vi "Complete Measurament RT.vi"() -> ()   [LabVIEW 2014]
uses:
  <vilib>/Platform/TimedLoop/XDataNode/timing_clust.ctl
  <vilib>/Platform/TimedLoop/XDataNode/nitl_modes.ctl
  <vilib>/Platform/TimedLoop/XDataNode/wakeup.ctl
  <vilib>/Analysis/Matrix/Datatypes/RealMatrix.ctl
  <vilib>/FPGAPlugInAG/sbRIO-9636/niLvFpga_Open_sbRIO-9636.vi
  <vilib>/rvi/interface/common/dynamic/niFpgaDynamicAddResources.vi
  <vilib>/FPGAPlugInAG/Dynamic/niLvFpga_Reset_Dynamic.vi
  <vilib>/Utility/error.llb/Error Cluster From Error Code.vi
  <vilib>/rvi/errors/niLvFpgaAdjustHostInterfaceError.vi
  <vilib>/rvi/interface/common/niFpgaWaitOnOcc.vi
  <vilib>/FPGAPlugInAG/Dynamic/niLvFpga_Run_Dynamic.vi
  <vilib>/FPGAPlugInAG/Dynamic/niLvFpga_Abort_Dynamic.vi
  <vilib>/FPGAPlugInAG/Dynamic/niLvFpga_Close_Dynamic.vi
  <vilib>/rvi/interface/nirviOpenFPGA/nirviOpenFPGA.xnode
  FPGA Bitfiles/LaserDistanceSen_FPGATarget_N-ParametricDoub_YVLbjAYtdP4.lvbitx
  FPGA Target/Test VIs/N-Parametric Double FFT Mesurament Test.vi
  FPGA Bitfiles/LaserDistanceSen_FPGATarget_N-ParametricDoub_qx5IM88U9d4.lvbitx
  FPGA Target/Test VIs/N-Parametric Double FFT Mesurament Test SLOW.vi
  <vilib>/rvi/interface/nirviMethod/nirviMethod.xnode
  <vilib>/rvi/interface/nirviReadWriteControl/nirviReadWriteControl.xnode
  <vilib>/Platform/TimedLoop/XDataNode/XDataNode.xnode
  <vilib>/rvi/interface/nirviCloseFPGA/nirviCloseFPGA.xnode
  <vilib>/FPGAPlugInAG/Dynamic/niLvFpga_ConfigureFifo_Dynamic.vi
  <vilib>/rvi/errors/niLvFpgaMergeErrorWithErrorCode.vi
  <vilib>/FPGAPlugInAG/Dynamic/niLvFpga_StartFifo_Dynamic.vi
  <vilib>/rvi/interface/Simulation/niFpgaSimulationCallBeginRW.vi
  <vilib>/FPGAPlugInAG/Dynamic/niLvFpga_ReadFifo_Dynamic.vi
  <vilib>/Platform/TimedLoop/XDataNode/XDNodeRunTimeDep.lvlib
  NiFpgaLv.dll
  <vilib>/Analysis/NI_AALBase.lvlib
  <vilib>/Analysis/Matrix/NI_Matrix.lvlib
panel:
  in  "Tab Control":enum32{"5 bin", "5 bin mean", "Distance "}(tab)
  out "5 bin FALL":T1(graph) caption="5 freq fall"
  out "5 bin RISE":T1(graph)
  out "5 bin mean/std FALL":T2(graph)
  in  "#meanBin":i32=100
  out "5 bin mean/std RISE":T2(graph)
  out "Distance and error":T1(graph)
  in  "Sample /Modulation Frequency":enum32{"40MHz/32KHz", "30MHz/24Khz"}(radio)
  in  "#movesignal":i32=10
  out "moving standard deviation rel":dbl format="%0.5f"
  out "moving mean":dbl format="%0.7f"
  out "StdDev Rel 1":dbl
  out "StdDev Rel 2":dbl
  out "Warning":bool
  out "Velocity (m/s)":dbl
  out "Distance (m)":dbl
  out "Mean Frequency":dbl
  out "Rise array size":i32
  out "Fall array size":i32
  out "Mean Frequency Rising (Hz)":dbl
  out "Mean Frequency Falling (Hz)":dbl
  in  "tieni premuto per":i32=1
  in  "Triangular Multiply Factor":dbl[](array[numeric])=[1.0, 0.8, 0.95, 0.85, 0.9]
  out "RISING Second Edge N-FFT":dbl[](graph)
  in  "Enable triangular scaling":bool=TRUE
  in  "Triangolo dritto?":bool
  out "FALLING First Edge N-FFT":dbl[](graph)
  in  "#Signals":u32(slide)=5 scale=1.0..5.0
  in  "stop":bool
  in  "Initial Latency points":u32(slide) scale=0.0..1249.0
  out "Elements Remaining FFT":u32
  out "Elements Remaining Signal":u32
  out "N-Signals":dbl[](graph)
  in  "Snapshot":bool
  in  "Windowing":T3(ring)=enum."Hanning"
  in  "first bin":i32=5
  in  "last bin":i32=255
  in  "lower limit 2":u32(slide)=738 scale=625.0..738.0
  in  "lower limit 1":u32(slide)=113 scale=0.0..113.0
  # "OFFLINE parameters"
  # "Max Detection FFT bin range"
  # "WARNING:\nOnce pressed wait untill the end of operation"
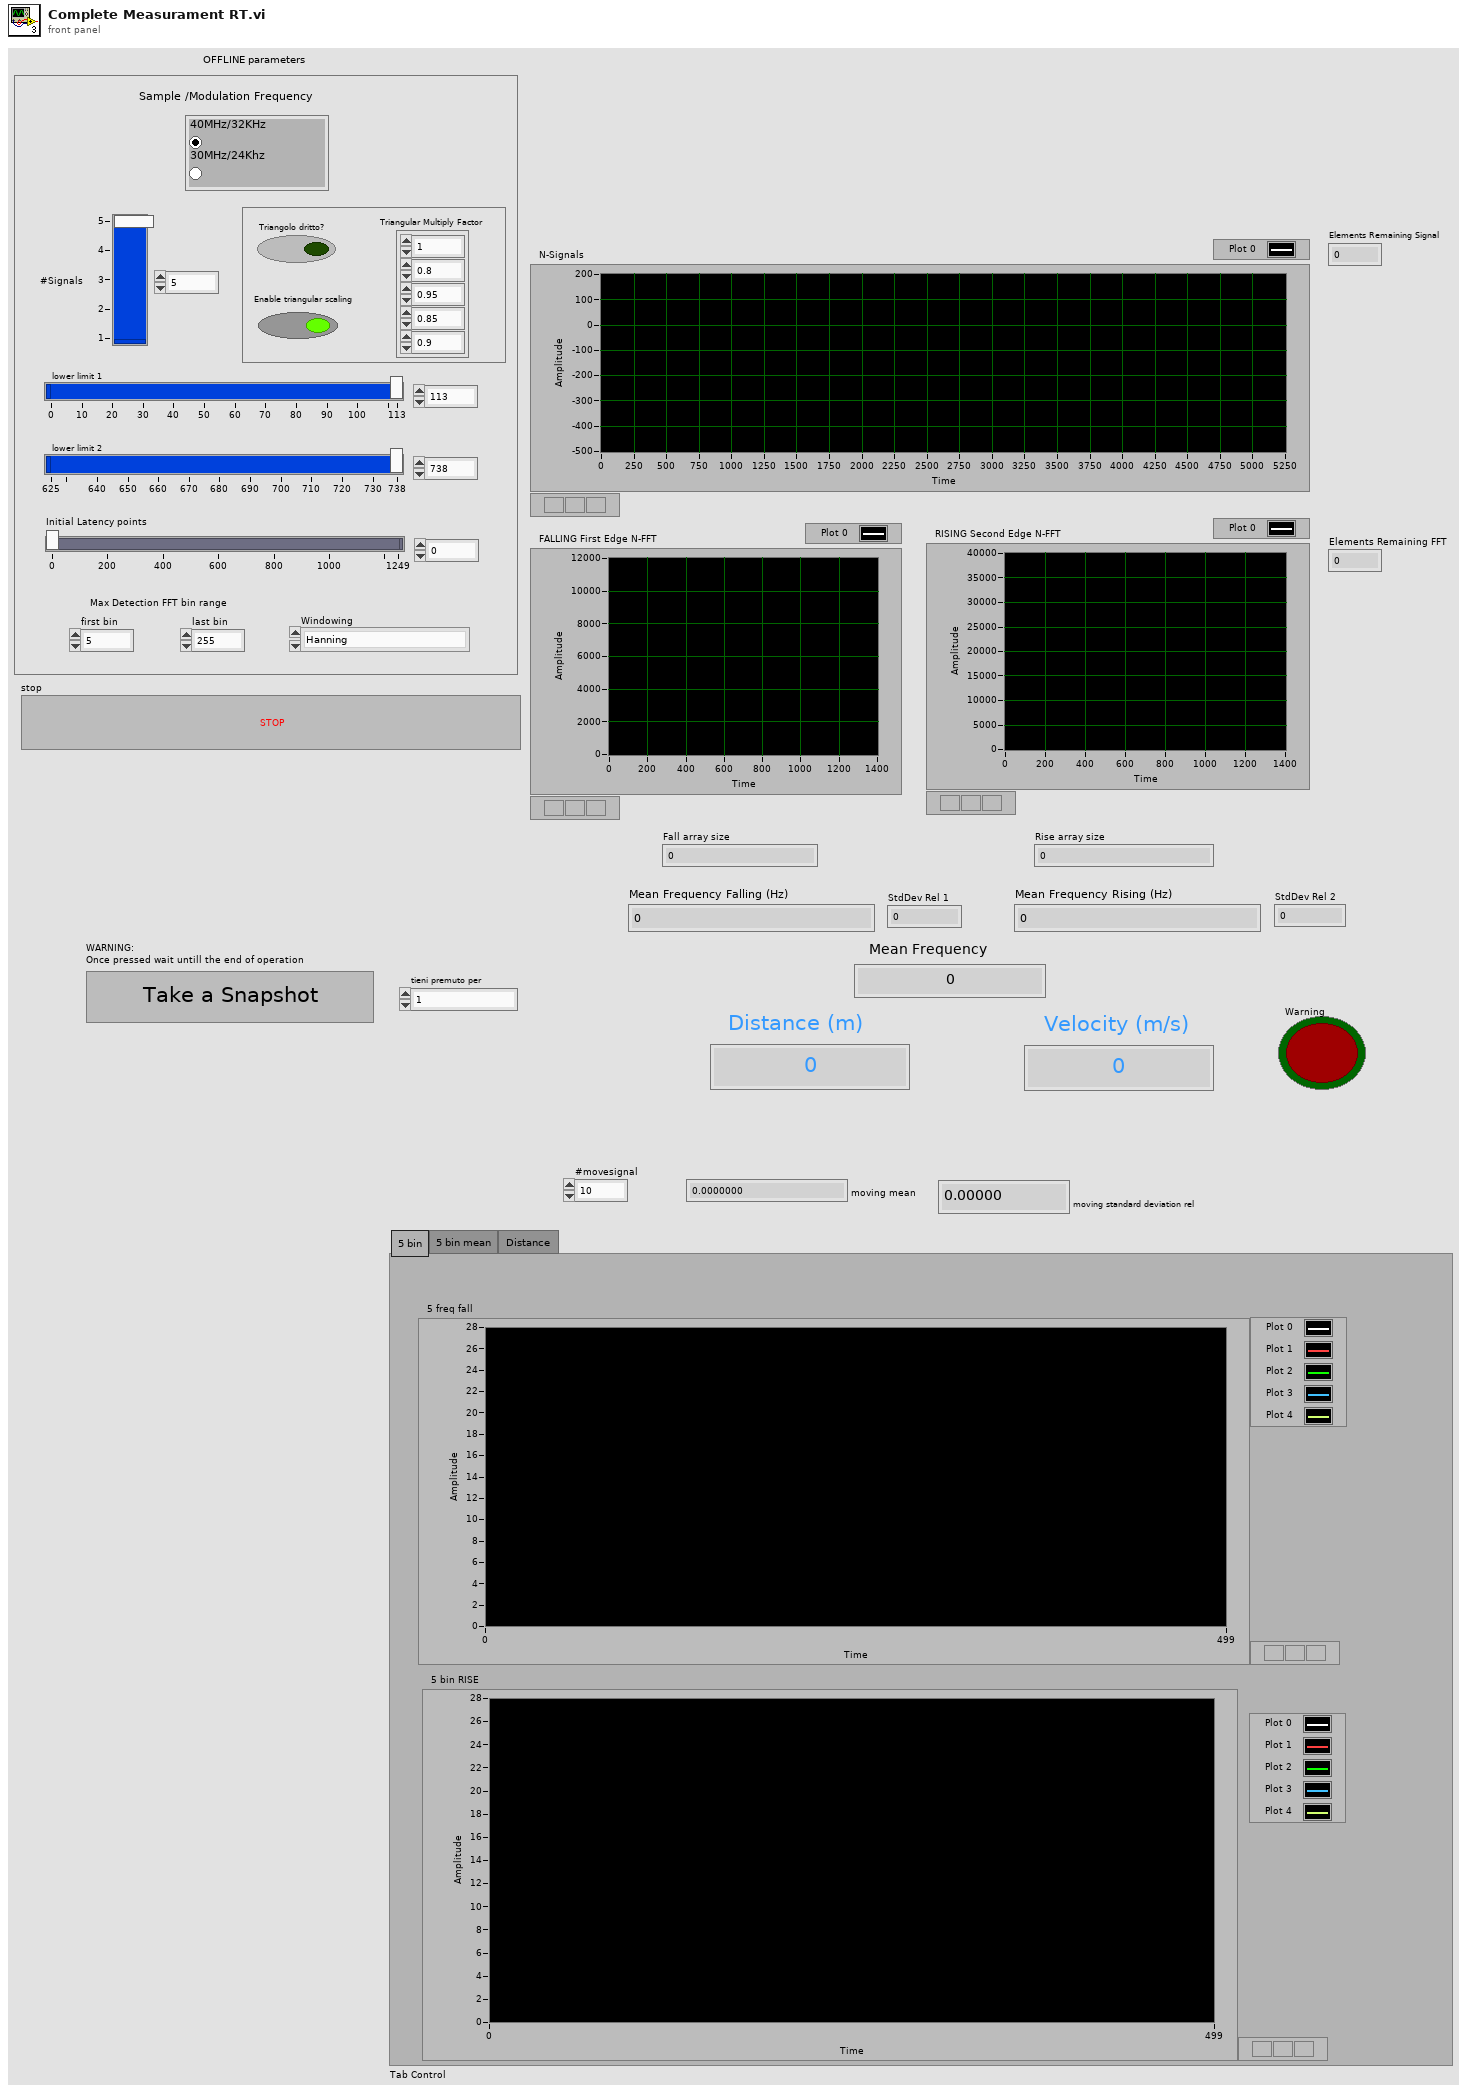
[diagram p1: front panel]
types:
  T1 = cluster{"[0]":dbl, "[1]":dbl, "[2]":dbl, "[3]":dbl, "[4]":dbl, "[5]":dbl, "[6]":dbl, "[7]":dbl, "[8]":dbl}
  T2 = cluster{"Array[0]":dbl, "Array[1]":dbl, "Array[2]":dbl, "Array[3]":dbl, "Array[4]":dbl, "Array[5]":dbl, "Array[6]":dbl, "Array[7]":dbl, "Array[8]":dbl}
  T3 = enum16{"None", "Hanning", "Hamming", "Blackman", "Blackman-Harris"}
  T4 = typedef "XDNodeRunTimeDep.lvlib/timing_clust.ctl" = cluster{"Expected End [f-1]":u64, "Actual End [f-1]":u64, "Finished Late? [f-1]":bool, "Expected End [i-1]":u64, "Actual End [i-1]":u64, "Finished Late? [i-1]":bool, "Expected Start [i]":u64, "Actual Start [i]":u64, "Expected Start [f]":u64, "Actual Start [f]":u64, "Source Name":string, "Structure Name":string, "Period":i64, "Deadline":i64, "Offset":i64, "Start":i64, "Priority":i32, "Timeout":i32, "Mode":T5, "Wakeup Reason":T6, "Error":errorcluster, "Source Type":string, "Secondary Source Type":string, "Global End Time":u64, "Global Start Time":u64, "Frame Duration":u64, "Iteration Duration":u64, "Assigned CPU":i32, "I/O Scan Engine Mode":u32}
  T5 = typedef "XDNodeRunTimeDep.lvlib/nitl_modes.ctl" = enum32{"No Change", "Process missed periods, maintain original phase", "Discard missed periods, maintain original phase", "Process missed periods, ignore original phase", "Discard missed periods, ignore original phase"}
  T6 = typedef "XDNodeRunTimeDep.lvlib/wakeup.ctl" = enum32{"Normal", "Aborted", "Asynchronous wakeup", "Timing source error", "Timed loop error", "Timeout"}
  T7 = typedef "NI_Matrix.lvlib/RealMatrix.ctl" = dbl[][]
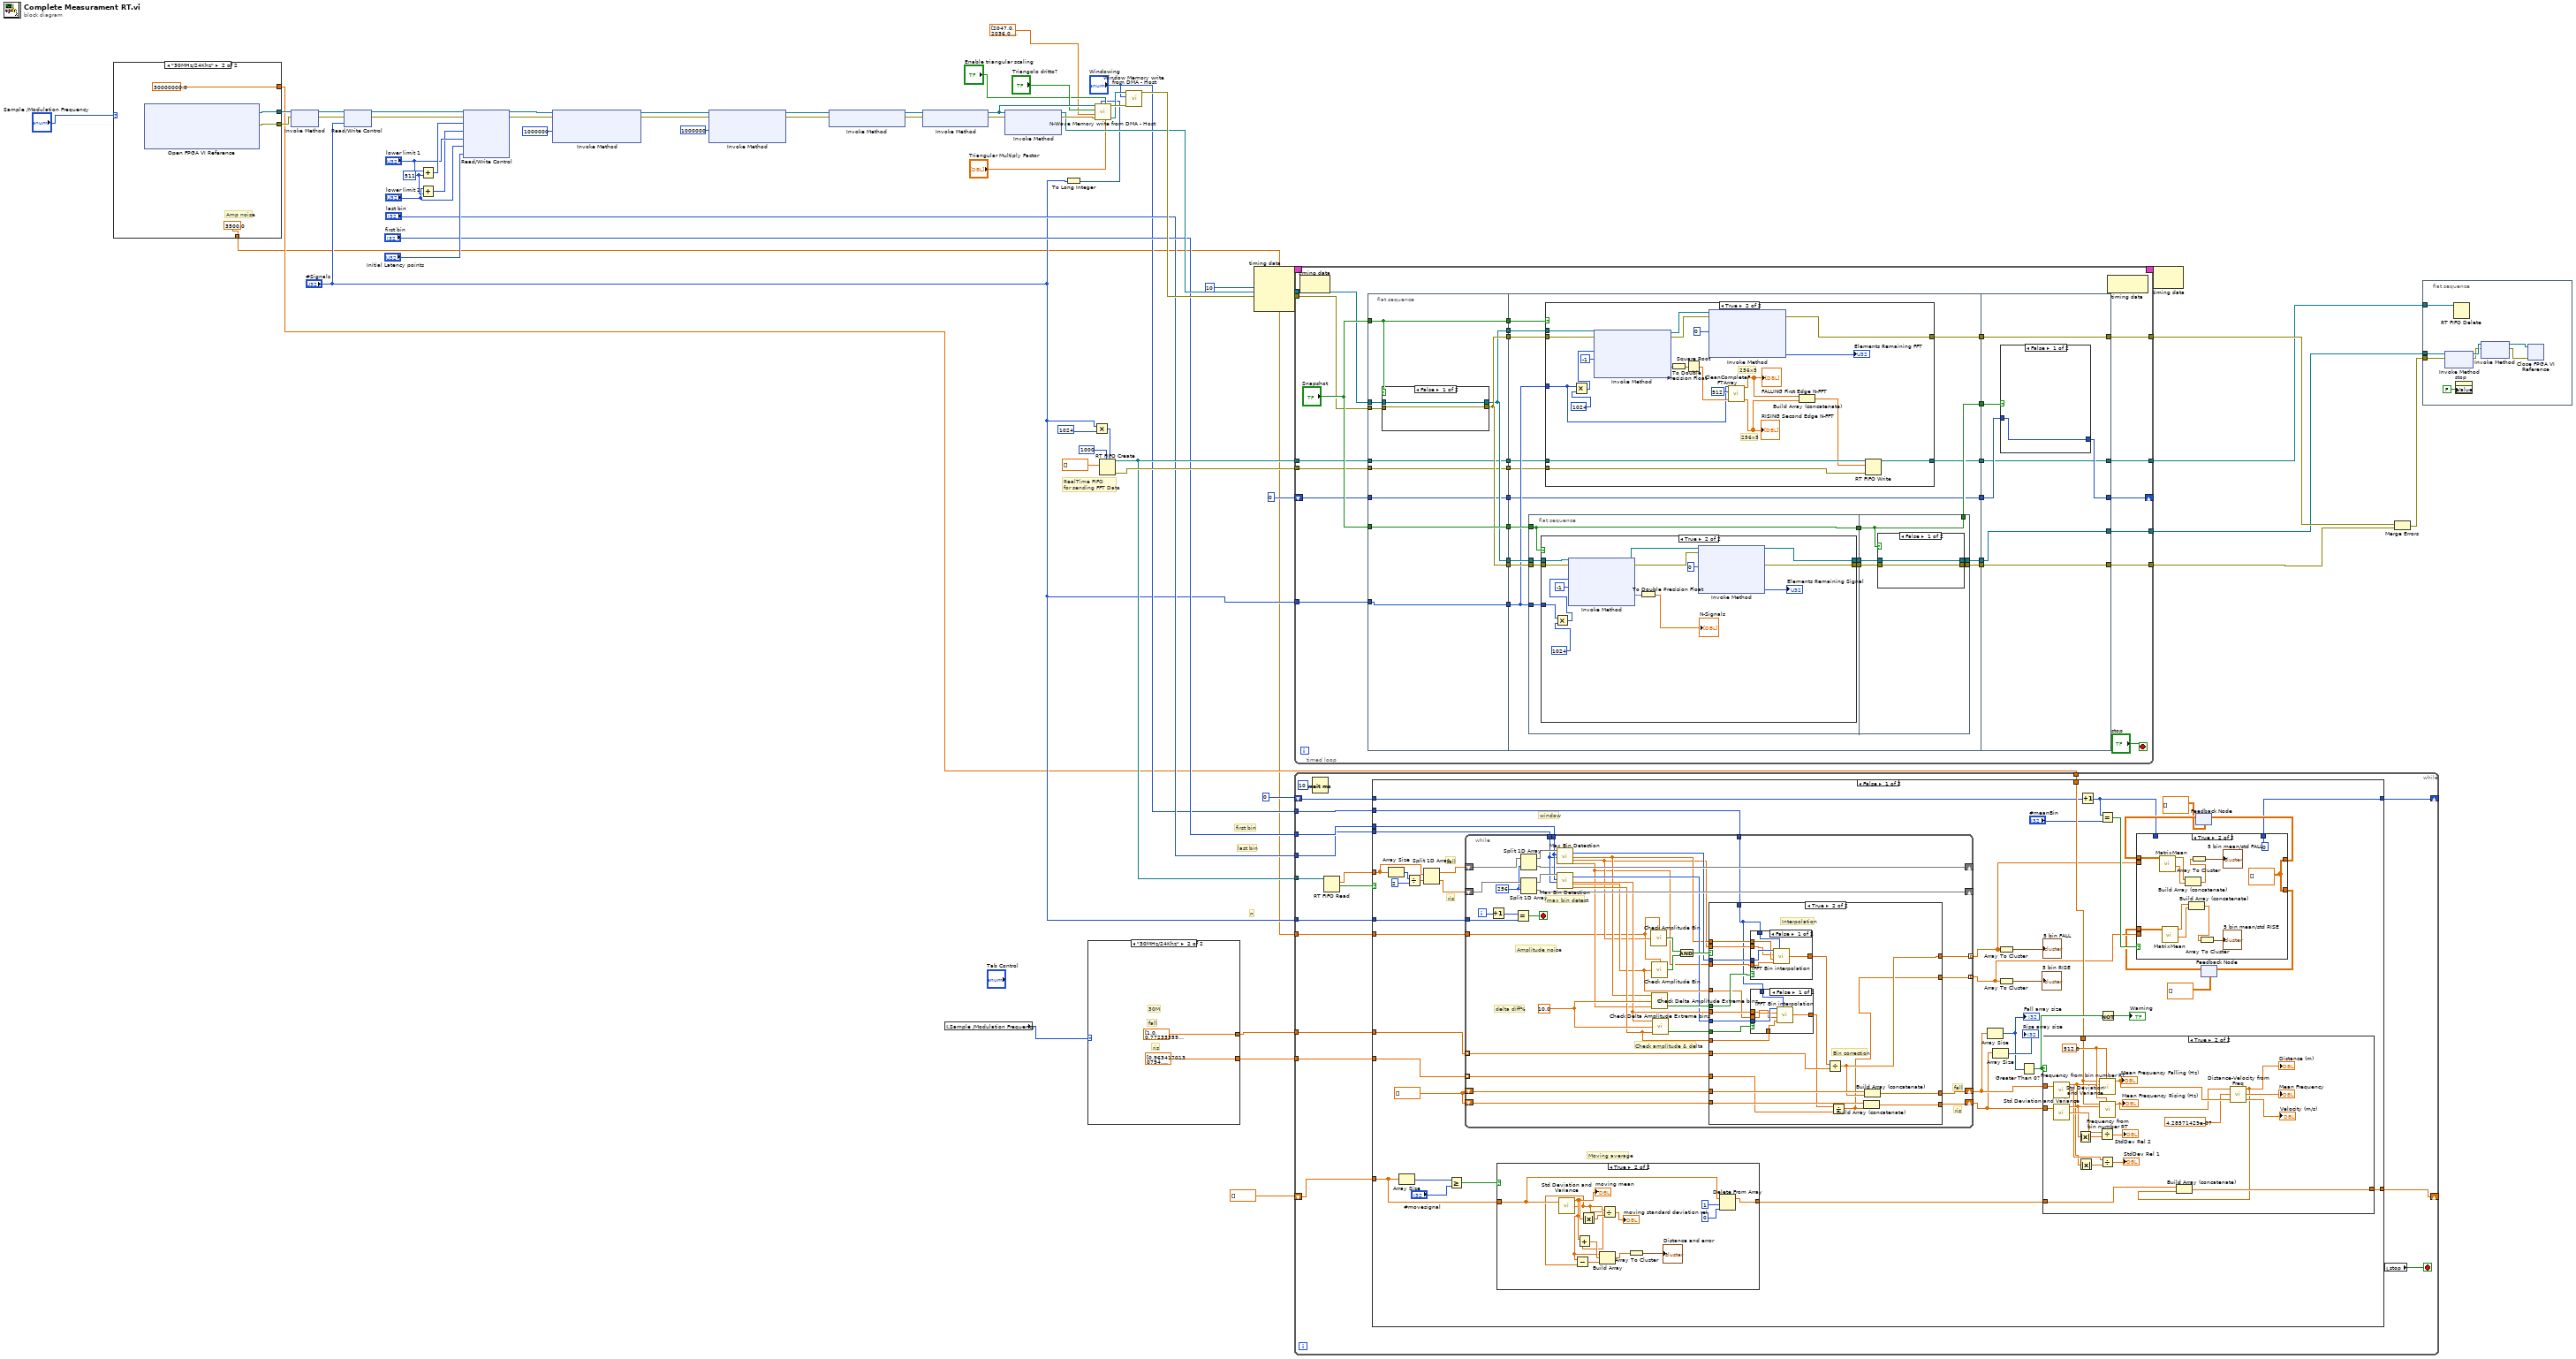
[diagram p0: block diagram]
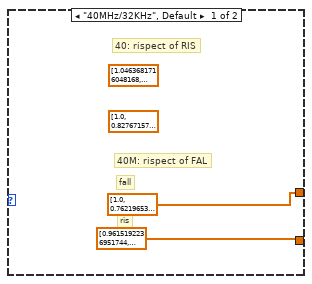
[diagram p2: hidden frame]
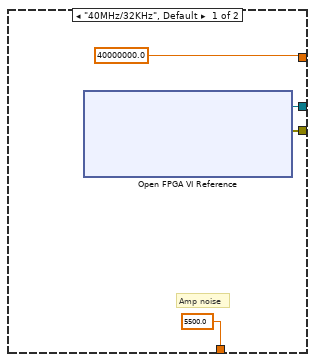
[diagram p3: hidden frame]
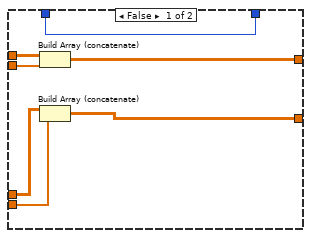
[diagram p4: hidden frame]
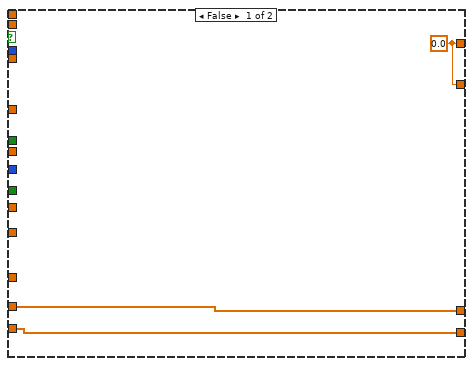
[diagram p7: hidden frame]
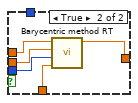
[diagram p8: hidden frame]
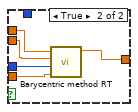
[diagram p9: hidden frame]
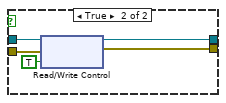
[diagram p11: hidden frame]
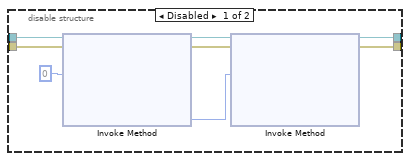
[diagram p13: hidden frame]
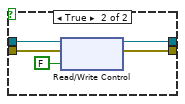
[diagram p14: hidden frame]
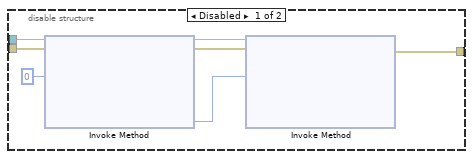
[diagram p16: hidden frame]
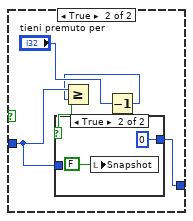
[diagram p17: hidden frame]
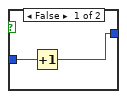
[diagram p18: hidden frame]
diagram:
  w57 = u32 511 ("y")
  # "n"
  # "last bin"
  # "first bin"
  # "RealTime FIFO \nfor sending FFT Data"
  n1 = case shown="\"30MHz/24Khz\"" "Sample /Modulation Frequency" {
    tunnel: [w65 w69] -> w31
    tunnel: [w64 w68] -> w30
    tunnel: [40000000.0 30000000.0] -> w6
    tunnel: [5500.0 ("Threshold Amp") 3500.0 ("Threshold Amp")] -> w1
    frame "40MHz/32KHz", Default {
      # "Amp noise"
      n2 = xnode "Open FPGA VI Reference"() -> ("FPGA VI Reference Out"=w65:refnum<k20>, "error out"=w64:errorcluster)  [unwired: 2 in]
    }
    frame "30MHz/24Khz" {
      # "Amp noise"
      n3 = xnode "Open FPGA VI Reference"() -> ("FPGA VI Reference Out"=w69:refnum<k20>, "error out"=w68:errorcluster)  [unwired: 2 in]
    }
  }
  n4 = xnode "Invoke Method"("FPGA VI Reference In"=w31, "error in"=w30) -> ("FPGA VI Reference Out"=w28:refnum<k20>, "error out"=w29:errorcluster)
  n5 = xnode "Read/Write Control"("FPGA VI Reference In"=w28, "error in"=w29, "n"="#Signals") -> ("FPGA VI Reference Out"=w27:refnum<k20>, "error out"=w26:errorcluster)
  n6 = Add(x="lower limit 1", y=w57) -> (x+y=w61:u32)
  n7 = Add(x="lower limit 2", y=w57) -> (x+y=w59:u32)
  n8 = xnode "Read/Write Control"("FPGA VI Reference In"=w27, "error in"=w26, "upper limit 1"=w61, "upper limit 2"=w59, "lower limit 1"="lower limit 1", "lower limit 2"="lower limit 2", "Latency points"="Initial Latency points") -> ("FPGA VI Reference Out"=w55:refnum<k20>, "error out"=w54:errorcluster)
  n9 = xnode "Invoke Method"("FPGA VI Reference In"=w55, "error in"=w54, "Requested Depth"=u32 1000000) -> ("FPGA VI Reference Out"=w42:refnum<k20>, "error out"=w43:errorcluster)  [unwired: 1 out]
  n10 = xnode "Invoke Method"("FPGA VI Reference In"=w42, "error in"=w43, "Requested Depth"=u32 1000000) -> ("FPGA VI Reference Out"=w49:refnum<k20>, "error out"=w50:errorcluster)  [unwired: 1 out]
  n11 = xnode "Invoke Method"("FPGA VI Reference In"=w49, "error in"=w50) -> ("FPGA VI Reference Out"=w40:refnum<k20>, "error out"=w41:errorcluster)
  n12 = xnode "Invoke Method"("FPGA VI Reference In"=w40, "error in"=w41) -> ("FPGA VI Reference Out"=w35:refnum<k20>, "error out"=w48:errorcluster)
  n13 = local read "Sample /Modulation Frequency"() -> (w3:enum32{"40MHz/32KHz", "30MHz/24Khz"})
  n14 = xnode "Invoke Method"("FPGA VI Reference In"=w35, "error in"=w48) -> ("FPGA VI Reference Out"=w36:refnum<k20>, "error out"=w39:errorcluster)  [unwired: 1 in]
  n15 = To Long Integer(number="#Signals") -> (32bit integer=w21:i32)
  n16 = case shown="\"30MHz/24Khz\"" w3 {
    tunnel: [dbl[] [1.0, 0.7621965374978185, 0.9584394857997629, 0.8264927572637538, 0.8956014637747813] ("mean factor 1") dbl[] [1.0, 0.7723335998303269, 0.9595435544705817, 0.8394441666056103, 0.8999330087703818] ("mean factor 1")] -> w5
    tunnel: [dbl[] [0.9615192236951744, 0.7991689735453839, 0.9195906148777597, 0.8398501694296071, 0.878805719221393] ("mean factor 2") dbl[] [0.9634170130794, 0.8025675631858347, 0.9199206430141584, 0.834350485116148, 0.8769354217012856] ("mean factor 2")] -> w4
    frame "40MHz/32KHz", Default {
      (unwired) dbl[] [1.0, 0.8276715727566772, 0.951057672906754, 0.8699894012780883, 0.9088749122499512] ("mean factor 2")
      (unwired) dbl[] [1.0463681716048168, 0.7798670577740541, 0.9941516729466621, 0.8518960261002109, 0.9344668620862013] ("mean factor 1")
      # "40: rispect of RIS"
      # "40M: rispect of FAL"
      # "ris"
      # "fall"
    }
    frame "30MHz/24Khz" {
      # "30M"
      # "ris"
      # "fall"
    }
  }
  n17 = Multiply(x="#Signals", y=u32 1024 ("elements in array (1)")) -> (x*y=w17:u32)
  n18 = call "N-Wave Memory write from DMA - Host.vi"("Triangular Multiply Factor"="Triangular Multiply Factor", "Enable triangular scaling"="Enable triangular scaling", "n"=w21, "error in"=w39, "Custom Triangular Signal (fal-ris)"=dbl[] [2047.0, 2036.0, 2024.0, 2013.0, 2002.0, 1990.0, 1979.0, 1968.0, 1956.0, 1945.0, 1934.0, 1923.0, 1912.0, 1900.0, 1889.0, 1878.0, 1867.0, 1856.0, 1845.0, 1833.0, 1822.0, 1811.0, 1800.0, 1789.0, 1778.0, 1767.0, 1756.0, 1745.0, 1734.0, 1723.0, 1712.0, 1702.0, 1691.0, 1680.0, 1669.0, 1658.0, 1647.0, 1636.0, 1626.0, 1615.0, 1604.0, 1593.0, 1583.0, 1572.0, 1561.0, 1550.0, 1540.0, 1529.0, 1518.0, 1508.0, 1497.0, 1487.0, 1476.0, 1465.0, 1455.0, 1444.0, 1434.0, 1423.0, 1413.0, 1402.0, 1392.0, 1381.0, 1371.0, 1360.0, 1350.0, 1340.0, 1329.0, 1319.0, 1309.0, 1298.0, 1288.0, 1278.0, 1267.0, 1257.0, 1247.0, 1237.0, 1226.0, 1216.0, 1206.0, 1196.0, 1186.0, 1176.0, 1165.0, 1155.0, 1145.0, 1135.0, 1125.0, 1115.0, 1105.0, 1095.0, 1085.0, 1075.0, 1065.0, 1055.0, 1045.0, 1035.0, 1025.0, 1015.0, 1006.0, 996.0, 986.0, 976.0, 966.0, 956.0, 947.0, 937.0, 927.0, 917.0, 908.0, 898.0, 888.0, 879.0, 869.0, 859.0, 850.0, 837.0, 826.0, 816.0, 804.0, 796.0, 788.0, 778.0, 769.0, 758.0, 750.0, 743.0, 733.0, 724.0, 717.0, 709.0, 701.0, 693.0, 686.0, 677.0, 669.0, 661.0, 653.0, 645.0, 638.0, 630.0, 622.0, 615.0, 607.0, 599.0, 592.0, 583.0, 576.0, 569.0, 561.0, 554.0, 547.0, 539.0, 532.0, 525.0, 518.0, 509.0, 501.0, 492.0, 486.0, 478.0, 471.0, 463.0, 456.0, 450.0, 442.0, 435.0, 429.0, 421.0, 415.0, 408.0, 401.0, 394.0, 388.0, 381.0, 375.0, 368.0, 361.0, 355.0, 349.0, 342.0, 336.0, 330.0, 323.0, 317.0, 311.0, 304.0, 298.0, 292.0, 286.0, 279.0, 273.0, 267.0, 261.0, 255.0, 249.0, 242.0, 236.0, 230.0, 224.0, 218.0, 212.0, 206.0, 200.0, 194.0, 187.0, 181.0, 175.0, 169.0, 163.0, 157.0, 150.0, 144.0, 138.0, 132.0, 125.0, 119.0, 113.0, 107.0, 101.0, 95.0, 88.0, 82.0, 77.0, 71.0, 65.0, 59.0, 53.0, 47.0, 41.0, 35.0, 29.0, 23.0, 18.0, 11.0, 6.0, 0.0, -6.0, -12.0, -18.0, -23.0, -29.0, -35.0, -41.0, -47.0, -52.0, -58.0, -64.0, -69.0, -75.0, -81.0, -87.0, -92.0, -98.0, -104.0, -109.0, -115.0, -121.0, -126.0, -132.0, -138.0, -144.0, -149.0, -155.0, -161.0, -166.0, -172.0, -177.0, -183.0, -189.0, -194.0, -200.0, -205.0, -211.0, -216.0, -222.0, -227.0, -233.0, -238.0, -244.0, -249.0, -255.0, -260.0, -266.0, -271.0, -277.0, -283.0, -288.0, -294.0, -299.0, -304.0, -310.0, -315.0, -321.0, -326.0, -331.0, -337.0, -342.0, -348.0, -353.0, -358.0, -364.0, -369.0, -375.0, -380.0, -385.0, -391.0, -396.0, -402.0, -407.0, -413.0, -418.0, -423.0, -429.0, -434.0, -439.0, -445.0, -450.0, -456.0, -461.0, -466.0, -472.0, -477.0, -483.0, -488.0, -493.0, -499.0, -504.0, -510.0, -515.0, -520.0, -526.0, -531.0, -537.0, -542.0, -548.0, -553.0, -558.0, -564.0, -569.0, -574.0, -580.0, -585.0, -590.0, -596.0, -601.0, -606.0, -612.0, -617.0, -622.0, -628.0, -633.0, -638.0, -644.0, -649.0, -654.0, -660.0, -665.0, -670.0, -676.0, -681.0, -686.0, -692.0, -697.0, -702.0, -708.0, -713.0, -718.0, -723.0, -729.0, -734.0, -739.0, -744.0, -750.0, -755.0, -760.0, -765.0, -771.0, -776.0, -781.0, -786.0, -792.0, -797.0, -802.0, -807.0, -812.0, -818.0, -823.0, -828.0, -833.0, -839.0, -844.0, -849.0, -854.0, -859.0, -865.0, -870.0, -875.0, -880.0, -885.0, -891.0, -896.0, -901.0, -906.0, -911.0, -916.0, -922.0, -927.0, -932.0, -937.0, -943.0, -948.0, -953.0, -958.0, -963.0, -969.0, -974.0, -979.0, -984.0, -989.0, -995.0, -1000.0, -1005.0, -1010.0, -1015.0, -1021.0, -1026.0, -1031.0, -1036.0, -1041.0, -1047.0, -1052.0, -1057.0, -1062.0, -1067.0, -1073.0, -1078.0, -1083.0, -1088.0, -1093.0, -1099.0, -1104.0, -1109.0, -1114.0, -1119.0, -1124.0, -1130.0, -1135.0, -1140.0, -1145.0, -1150.0, -1156.0, -1161.0, -1166.0, -1171.0, -1176.0, -1182.0, -1187.0, -1192.0, -1197.0, -1202.0, -1207.0, -1213.0, -1218.0, -1223.0, -1228.0, -1233.0, -1238.0, -1244.0, -1249.0, -1254.0, -1259.0, -1264.0, -1269.0, -1275.0, -1280.0, -1285.0, -1290.0, -1295.0, -1300.0, -1305.0, -1311.0, -1316.0, -1321.0, -1326.0, -1331.0, -1336.0, -1342.0, -1347.0, -1352.0, -1357.0, -1362.0, -1367.0, -1372.0, -1378.0, -1383.0, -1388.0, -1393.0, -1398.0, -1403.0, -1408.0, -1414.0, -1419.0, -1424.0, -1429.0, -1434.0, -1439.0, -1444.0, -1450.0, -1455.0, -1460.0, -1465.0, -1470.0, -1475.0, -1480.0, -1486.0, -1491.0, -1496.0, -1501.0, -1506.0, -1511.0, -1516.0, -1522.0, -1527.0, -1532.0, -1537.0, -1542.0, -1547.0, -1552.0, -1558.0, -1563.0, -1568.0, -1573.0, -1578.0, -1583.0, -1588.0, -1593.0, -1599.0, -1604.0, -1609.0, -1614.0, -1619.0, -1624.0, -1629.0, -1634.0, -1640.0, -1645.0, -1650.0, -1655.0, -1660.0, -1665.0, -1670.0, -1675.0, -1681.0, -1686.0, -1691.0, -1696.0, -1701.0, -1706.0, -1711.0, -1716.0, -1722.0, -1727.0, -1732.0, -1737.0, -1742.0, -1747.0, -1752.0, -1757.0, -1762.0, -1768.0, -1773.0, -1778.0, -1783.0, -1788.0, -1793.0, -1798.0, -1803.0, -1808.0, -1814.0, -1819.0, -1824.0, -1829.0, -1834.0, -1839.0, -1844.0, -1849.0, -1854.0, -1859.0, -1865.0, -1870.0, -1875.0, -1880.0, -1885.0, -1890.0, -1895.0, -1900.0, -1905.0, -1911.0, -1916.0, -1921.0, -1926.0, -1931.0, -1936.0, -1941.0, -1946.0, -1951.0, -1956.0, -1961.0, -1967.0, -1972.0, -1977.0, -1982.0, -1987.0, -1992.0, -1997.0, -2002.0, -2007.0, -2012.0, -2017.0, -2023.0, -2028.0, -2033.0, -2038.0, -2043.0, -2048.0, -2047.0, -2034.0, -2021.0, -2009.0, -1996.0, -1983.0, -1970.0, -1957.0, -1945.0, -1932.0, -1919.0, -1907.0, -1894.0, -1881.0, -1869.0, -1856.0, -1844.0, -1831.0, -1819.0, -1806.0, -1794.0, -1781.0, -1769.0, -1757.0, -1744.0, -1732.0, -1719.0, -1707.0, -1695.0, -1682.0, -1670.0, -1658.0, -1646.0, -1634.0, -1621.0, -1609.0, -1597.0, -1585.0, -1573.0, -1561.0, -1549.0, -1537.0, -1525.0, -1513.0, -1501.0, -1489.0, -1477.0, -1465.0, -1453.0, -1441.0, -1429.0, -1417.0, -1405.0, -1394.0, -1382.0, -1370.0, -1358.0, -1347.0, -1335.0, -1323.0, -1312.0, -1300.0, -1288.0, -1277.0, -1265.0, -1254.0, -1242.0, -1231.0, -1219.0, -1208.0, -1196.0, -1185.0, -1173.0, -1162.0, -1150.0, -1139.0, -1128.0, -1116.0, -1105.0, -1094.0, -1083.0, -1071.0, -1060.0, -1049.0, -1038.0, -1027.0, -1015.0, -1004.0, -993.0, -982.0, -971.0, -960.0, -949.0, -938.0, -927.0, -916.0, -905.0, -894.0, -883.0, -873.0, -862.0, -851.0, -840.0, -829.0, -819.0, -808.0, -797.0, -786.0, -776.0, -765.0, -754.0, -744.0, -733.0, -722.0, -712.0, -697.0, -685.0, -674.0, -661.0, -652.0, -643.0, -632.0, -622.0, -610.0, -602.0, -594.0, -583.0, -574.0, -566.0, -558.0, -550.0, -542.0, -534.0, -525.0, -516.0, -507.0, -499.0, -491.0, -483.0, -475.0, -467.0, -459.0, -451.0, -443.0, -435.0, -426.0, -419.0, -411.0, -404.0, -396.0, -388.0, -381.0, -373.0, -366.0, -359.0, -349.0, -341.0, -331.0, -325.0, -317.0, -309.0, -301.0, -295.0, -288.0, -280.0, -273.0, -266.0, -259.0, -252.0, -246.0, -239.0, -231.0, -225.0, -219.0, -212.0, -205.0, -199.0, -192.0, -186.0, -180.0, -173.0, -167.0, -161.0, -155.0, -148.0, -142.0, -136.0, -130.0, -124.0, -118.0, -112.0, -106.0, -100.0, -94.0, -88.0, -82.0, -76.0, -70.0, -64.0, -58.0, -52.0, -46.0, -40.0, -34.0, -28.0, -21.0, -15.0, -9.0, -3.0, 2.0, 9.0, 15.0, 21.0, 27.0, 33.0, 39.0, 45.0, 51.0, 57.0, 63.0, 69.0, 75.0, 81.0, 86.0, 92.0, 98.0, 103.0, 110.0, 116.0, 121.0, 127.0, 133.0, 138.0, 144.0, 149.0, 155.0, 161.0, 166.0, 172.0, 177.0, 183.0, 189.0, 194.0, 200.0, 205.0, 211.0, 216.0, 221.0, 227.0, 232.0, 238.0, 243.0, 249.0, 254.0, 259.0, 265.0, 270.0, 276.0, 281.0, 286.0, 292.0, 297.0, 303.0, 308.0, 314.0, 319.0, 324.0, 329.0, 335.0, 340.0, 345.0, 351.0, 356.0, 361.0, 366.0, 371.0, 377.0, 382.0, 387.0, 392.0, 397.0, 403.0, 408.0, 413.0, 418.0, 423.0, 429.0, 434.0, 439.0, 444.0, 449.0, 454.0, 459.0, 464.0, 469.0, 474.0, 479.0, 484.0, 489.0, 494.0, 499.0, 504.0, 509.0, 514.0, 520.0, 525.0, 530.0, 535.0, 540.0, 545.0, 550.0, 555.0, 560.0, 565.0, 570.0, 575.0, 580.0, 585.0, 590.0, 595.0, 600.0, 605.0, 610.0, 615.0, 620.0, 625.0, 630.0, 636.0, 641.0, 646.0, 651.0, 656.0, 661.0, 666.0, 671.0, 676.0, 681.0, 686.0, 691.0, 696.0, 701.0, 706.0, 711.0, 716.0, 721.0, 726.0, 731.0, 736.0, 741.0, 746.0, 751.0, 756.0, 761.0, 765.0, 770.0, 775.0, 780.0, 785.0, 790.0, 795.0, 800.0, 805.0, 810.0, 815.0, 820.0, 825.0, 829.0, 834.0, 839.0, 844.0, 849.0, 854.0, 859.0, 864.0, 868.0, 873.0, 878.0, 883.0, 888.0, 893.0, 897.0, 902.0, 907.0, 912.0, 917.0, 921.0, 926.0, 931.0, 936.0, 941.0, 945.0, 950.0, 955.0, 960.0, 965.0, 969.0, 974.0, 979.0, 984.0, 988.0, 993.0, 998.0, 1003.0, 1007.0, 1012.0, 1017.0, 1022.0, 1027.0, 1031.0, 1036.0, 1041.0, 1046.0, 1051.0, 1055.0, 1060.0, 1065.0, 1070.0, 1075.0, 1079.0, 1084.0, 1089.0, 1094.0, 1098.0, 1103.0, 1108.0, 1113.0, 1118.0, 1122.0, 1127.0, 1132.0, 1137.0, 1141.0, 1146.0, 1151.0, 1156.0, 1161.0, 1165.0, 1170.0, 1175.0, 1180.0, 1184.0, 1189.0, 1194.0, 1199.0, 1204.0, 1208.0, 1213.0, 1218.0, 1223.0, 1227.0, 1232.0, 1237.0, 1242.0, 1246.0, 1251.0, 1256.0, 1261.0, 1265.0, 1270.0, 1275.0, 1280.0, 1284.0, 1289.0, 1294.0, 1299.0, 1303.0, 1308.0, 1313.0, 1318.0, 1322.0, 1327.0, 1332.0, 1336.0, 1341.0, 1346.0, 1351.0, 1355.0, 1360.0, 1365.0, 1370.0, 1374.0, 1379.0, 1384.0, 1388.0, 1393.0, 1398.0, 1403.0, 1407.0, 1412.0, 1417.0, 1421.0, 1426.0, 1431.0, 1436.0, 1440.0, 1445.0, 1450.0, 1454.0, 1459.0, 1464.0, 1469.0, 1473.0, 1478.0, 1483.0, 1487.0, 1492.0, 1497.0, 1502.0, 1506.0, 1511.0, 1516.0, 1520.0, 1525.0, 1530.0, 1535.0, 1539.0, 1544.0, 1549.0, 1553.0, 1558.0, 1563.0, 1567.0, 1572.0, 1577.0, 1582.0, 1586.0, 1591.0, 1596.0, 1600.0, 1605.0, 1610.0, 1614.0, 1619.0, 1624.0, 1628.0, 1633.0, 1638.0, 1643.0, 1647.0, 1652.0, 1657.0, 1661.0, 1666.0, 1671.0, 1675.0, 1680.0, 1685.0, 1689.0, 1694.0, 1699.0, 1703.0, 1708.0, 1713.0, 1717.0, 1722.0, 1727.0, 1731.0, 1736.0, 1741.0, 1746.0, 1750.0, 1755.0, 1760.0, 1764.0, 1769.0, 1774.0, 1778.0, 1783.0, 1788.0, 1792.0, 1797.0, 1802.0, 1806.0, 1811.0, 1816.0, 1820.0, 1825.0, 1830.0, 1834.0, 1839.0, 1844.0, 1848.0, 1853.0, 1858.0, 1862.0, 1867.0, 1871.0, 1876.0, 1881.0, 1885.0, 1890.0, 1895.0, 1899.0, 1904.0, 1909.0, 1913.0, 1918.0, 1923.0, 1927.0, 1932.0, 1937.0, 1941.0, 1946.0, 1951.0, 1955.0, 1960.0, 1965.0, 1969.0, 1974.0, 1978.0, 1983.0, 1988.0, 1992.0, 1997.0, 2002.0, 2006.0, 2011.0, 2016.0, 2020.0, 2025.0, 2029.0, 2034.0, 2039.0, 2043.0, 2048.0] ("Complete SkewTri"), "Triangolo dritto?"="Triangolo dritto?", "FPGA VI Reference In"=w35) -> ("FPGA VI Reference Out"=w37:refnum<k20>, "error out"=w38:errorcluster)  [unwired: 2 in, 1 out]
  n19 = RT FIFO Create(1:dbl[] [] ("double precision float"), 4:u32 1000 ("size (10)"), 6:w17) -> (8:w14:refnum<k33>, 11:w15:errorcluster)  [unwired: 5 in, 1 out]
  n20 = call "Window Memory write from DMA - Host.vi"("error in"=w38, "Enum"="Windowing", "FPGA VI Reference In"=w37) -> ("error out"=w56:errorcluster)  [unwired: 5 in, 3 out]
  n21 = node-c288(i64 10 ("Period")) -> (w34:T4)  [unwired: 3 in]
  n22 = while {
    tunnel: w14 -> [w89]
    tunnel: "first bin" -> [w86]
    tunnel: "last bin" -> [w85]
    tunnel: "Windowing" -> [w84]
    tunnel: "#Signals" -> [w83]
    shift-right: [w80] -> _
    shift-left: dbl[] [] ("appended array") -> [w81]
    tunnel: w6 -> [w79]
    tunnel: w5 -> [w78]
    tunnel: w4 -> [w77]
    shift-right: [w75] -> _
    shift-left: 0 ("first bin") -> [w76]
    tunnel: w1 -> [w74]
    stop <- w82 stop-if-true
    n23 = Wait (ms)(milliseconds to wait=u32 10 ("millisecond multiple")) -> ()  [unwired: 1 out]
    n24 = RT FIFO Read(0:w89) -> (9:w87:dbl[], 10:w88:bool)  [unwired: 3 in, 3 out]
    n25 = case shown="False" w88 {
      tunnel: w87 -> [w132 _]
      tunnel: w86 -> [w128 _]
      tunnel: w85 -> [w127 _]
      tunnel: w84 -> [w126 _]
      tunnel: w83 -> [w123 _]
      tunnel: w81 -> [w112 w270]
      tunnel: [w110 w270] -> w80
      tunnel: w79 -> [w107 _]
      tunnel: w78 -> [w106 _]
      tunnel: w77 -> [w105 _]
      tunnel: w76 -> [w104 w269]
      tunnel: [w92 w269] -> w75
      tunnel: w74 -> [w91 _]
      frame False {
        w122 = dbl[] [] ("appended array")
        # "Moving average"
        # "window"
        # "ris"
        # "fall"
        n26 = Array Size(array=w132) -> (size(s)=w130:i32)
        n27 = Array Size(array=w112) -> (size(s)=w115:i32)
        n28 = Divide(x=w130, y=2) -> (x/y=w131:dbl)
        n29 = Split 1D Array(array=w132, index=w131) -> (first subarray=w124:dbl[], second subarray=w125:dbl[])
        n30 = Greater Or Equal?(x=w115, y="#movesignal") -> (x >= y?=w114:bool)
        n31 = while {
          shift-right: [w210] -> _
          shift-left: w124 -> [w222]
          shift-right: [w211] -> _
          shift-left: w125 -> [w221]
          tunnel: w128 -> [w218]
          tunnel: w127 -> [w217]
          tunnel: w126 -> [w195]
          tunnel: w123 -> [w215]
          shift-right: [w194] -> w121
          shift-left: w122 -> [w192]
          shift-right: [w193] -> w120
          shift-left: w122 -> [w191]
          tunnel: w106 -> [w190] mode=indexing
          tunnel: w105 -> [w189] mode=indexing
          tunnel: [w188] -> w102 mode=indexing
          tunnel: [w187] -> w100 mode=indexing
          tunnel: w91 -> [w186]
          i -> [w212]
          stop <- w216 stop-if-true
          w209 = 10.0 ("Max Difference %")
          w214 = 256 ("x")
          # "delta diff%"
          # "ris"
          # "fall"
          # "max bin detect"
          # "Check amplitude & delta"
          # "Amplitude noise"
          n32 = Increment(x=w212) -> (x+1=w213:i32)
          n33 = Equal?(x=w213, y=w215) -> (x = y?=w216:bool)
          n34 = Split 1D Array(array=w222, index=w214) -> (first subarray=w220:dbl[], second subarray=w210:dbl[])
          n35 = Split 1D Array(array=w221, index=w214) -> (first subarray=w219:dbl[], second subarray=w211:dbl[])
          n36 = call "Max Bin Detection.vi"("FFT Array"=w220, "Init Discard Bins"=w218, "Last Discard Bins"=w217) -> ("Max Bin"=w199:i32, "Prev Max Amp"=w198:dbl, "Max Amp"=w197:dbl, "Succ Max Amp"=w196:dbl)  [unwired: 11 in, 2 out]
          n37 = call "Max Bin Detection.vi"("FFT Array"=w219, "Init Discard Bins"=w218, "Last Discard Bins"=w217) -> ("Max Bin"=w200:i32, "Prev Max Amp"=w203:dbl, "Max Amp"=w201:dbl, "Succ Max Amp"=w202:dbl)  [unwired: 11 in, 2 out]
          n38 = call "Check Amplitude Bin.vi"("Threshold Amp"=w186, "Max Amp"=w197) -> ("Check Amp Ok?"=w208:bool)  [unwired: 2 in]
          n39 = call "Check Amplitude Bin.vi"("Threshold Amp"=w186, "Max Amp"=w201) -> ("Check Amp Ok?"=w207:bool)  [unwired: 2 in]
          n40 = call "Check Delta Amplitude Extreme bins.vi"("Succ Max Amp"=w196, "Max Difference %"=w209, "Prev Max Amp"=w198) -> ("Check Delta Amp Ok?"=w205:bool)  [unwired: 1 in, 1 out]
          n41 = call "Check Delta Amplitude Extreme bins.vi"("Succ Max Amp"=w202, "Max Difference %"=w209, "Prev Max Amp"=w203) -> ("Check Delta Amp Ok?"=w204:bool)  [unwired: 1 in, 1 out]
          n42 = And(x=w208, y=w207) -> (x .and. y?=w206:bool)
          n43 = case shown="True" w206 {
            tunnel: w205 -> [_ w246]
            tunnel: w204 -> [_ w245]
            tunnel: w203 -> [_ w244]
            tunnel: w202 -> [_ w243]
            tunnel: w201 -> [_ w242]
            tunnel: w200 -> [_ w241]
            tunnel: w199 -> [_ w240]
            tunnel: w198 -> [_ w239]
            tunnel: w197 -> [_ w238]
            tunnel: w196 -> [_ w237]
            tunnel: w195 -> [_ w236]
            tunnel: [w225 w231] -> w194
            tunnel: [w224 w230] -> w193
            tunnel: w192 -> [w225 w235]
            tunnel: w191 -> [w224 w234]
            tunnel: w190 -> [_ w233]
            tunnel: w189 -> [_ w232]
            tunnel: [w223 w227] -> w188
            tunnel: [w223 w226] -> w187
            frame False {
              w223 = 0.0
            }
            frame True {
              # "Bin correction"
              # "Interpolation"
              n44 = case shown="False" w246 {
                tunnel: w240 -> [w262 w268]
                tunnel: w239 -> [w260 w267]
                tunnel: w238 -> [w259 w266]
                tunnel: w237 -> [w258 w265]
                tunnel: [w261 w264] -> w229
                tunnel: w236 -> [w263 _]
                frame False {
                  n45 = call "IFFT Bin interpolation.vi"("Max Bin"=w262, "Max Amp"=w259, "Prev Max Amp"=w260, "Succ Max Amp"=w258, "Windowing"=w263) -> ("Interpolate Bin"=w261:dbl)
                }
                frame True {
                  n46 = call "Barycentric method RT.vi"("Next Amp"=w265, "Max Bin"=w268, "Max Amp"=w266, "Prev Amp"=w267) -> ("Bin"=w264:dbl)  [unwired: 7 in]
                }
              }
              n47 = case shown="False" w245 {
                tunnel: w244 -> [w248 w257]
                tunnel: w243 -> [w247 w256]
                tunnel: w242 -> [w249 w255]
                tunnel: w241 -> [w251 w254]
                tunnel: [w250 w253] -> w228
                tunnel: w236 -> [w252 _]
                frame False {
                  n48 = call "IFFT Bin interpolation.vi"("Max Bin"=w251, "Max Amp"=w249, "Prev Max Amp"=w248, "Succ Max Amp"=w247, "Windowing"=w252) -> ("Interpolate Bin"=w250:dbl)
                }
                frame True {
                  n49 = call "Barycentric method RT.vi"("Next Amp"=w256, "Max Bin"=w254, "Max Amp"=w255, "Prev Amp"=w257) -> ("Bin"=w253:dbl)  [unwired: 7 in]
                }
              }
              n50 = Divide(x=w229, y=w233) -> (x/y=w227:dbl)
              n51 = Divide(x=w228, y=w232) -> (x/y=w226:dbl)
              n52 = Build Array (concatenate)(w234, w226) -> (w230:dbl[])
              n53 = Build Array (concatenate)(w235, w227) -> (w231:dbl[])
            }
          }
        }
        n54 = case shown="True" w114 {
          tunnel: w112 -> [w152 w162]
          tunnel: [w152 w159] -> w111
          frame False {
          }
          frame True {
            n55 = call <vilib>:"Std Deviation and Variance.vi"("X"=w162) -> ("mean"=w155:dbl, "standard deviation"=w154:dbl)  [unwired: 1 in, 1 out]
            "moving mean" <- w155
            n56 = Subtract(x=w155, y=w154) -> (x-y=w156:dbl)
            n57 = Add(x=w155, y=w154) -> (x+y=w157:dbl)
            n58 = Absolute Value(x=w155) -> (abs(x)=w164:dbl)
            n59 = Build Array(w155, w157, w156) -> (w158:dbl[])
            n60 = Divide(x=w154, y=w164) -> (x/y=→"moving standard deviation rel":dbl)
            n61 = Array To Cluster(array=w158) -> (cluster=→"Distance and error":T1)
            n62 = Delete From Array(array=w162, length=1, index=0) -> (array with subset deleted=w159:dbl[])  [unwired: 1 out]
          }
        }
        n63 = Array Size(array=w121) -> (size(s)=w118:i32)
        "Fall array size" <- w118
        n64 = Array Size(array=w120) -> (size(s)=→"Rise array size":i32)
        n65 = Array To Cluster(array=w102) -> (cluster=→"5 bin FALL":T1)
        n66 = Array To Cluster(array=w100) -> (cluster=→"5 bin RISE":T1)
        n67 = Greater Than 0?(x=w118) -> (x > 0?=w116:bool)
        n68 = case shown="True" w116 {
          tunnel: w121 -> [_ w184]
          tunnel: w120 -> [_ w183]
          tunnel: w111 -> [w165 w169]
          tunnel: [w165 w168] -> w110
          tunnel: w107 -> [_ w167]
          frame False {
          }
          frame True {
            w185 = 512.0 ("FFT size")
            n69 = call <vilib>:"Std Deviation and Variance.vi"("X"=w184) -> ("mean"=w170:dbl, "standard deviation"=w171:dbl)  [unwired: 1 in, 1 out]
            n70 = call <vilib>:"Std Deviation and Variance.vi"("X"=w183) -> ("mean"=w175:dbl, "standard deviation"=w177:dbl)  [unwired: 1 in, 1 out]
            n71 = Absolute Value(x=w175) -> (abs(x)=w176:dbl)
            n72 = Absolute Value(x=w170) -> (abs(x)=w172:dbl)
            n73 = call "Frequency from bin number RT.vi"("FFT size"=w185, "Bin number"=w170, "Sample Rate (S/s)"=w167) -> ("Detected Frequency (Hz)"=w182:dbl)  [unwired: 8 in]
            "Mean Frequency Falling (Hz)" <- w182
            n74 = Divide(x=w177, y=w176) -> (x/y=→"StdDev Rel 2":dbl)
            n75 = call "Frequency from bin number RT.vi"("FFT size"=w185, "Bin number"=w175, "Sample Rate (S/s)"=w167) -> ("Detected Frequency (Hz)"=w181:dbl)  [unwired: 8 in]
            "Mean Frequency Rising (Hz)" <- w181
            n76 = Divide(x=w171, y=w172) -> (x/y=→"StdDev Rel 1":dbl)
            n77 = call "Distance-Velocity from Freq.vi"("freq_rising"=w181, "Empirical Distance Costant"=4.28571429e-07, "freq_falling"=w182) -> ("Distance (m)"=w166:dbl, "Mean Frequency"=→"Mean Frequency":dbl, "Velocity (m/s)"=→"Velocity (m/s)":dbl)  [unwired: 2 in]
            "Distance (m)" <- w166
            n78 = Build Array (concatenate)(w169, w166) -> (w168:dbl[])
          }
        }
        n79 = Increment(x=w104) -> (x+1=w93:i32)
        n80 = Equal?(x=w93, y="#meanBin") -> (x = y?=w103:bool)
        n81 = Not(x=w116) -> (.not. x?=→"Warning":bool)
        n82 = feedback #1(T7 [] ("Real Matrix")) -> (w98:T7)
        n83 = feedback #2(T7 [] ("Real Matrix")) -> (w96:T7)
        n84 = case shown="True" w103 {
          tunnel: w100 -> [w138 _]
          tunnel: w102 -> [w139 _]
          tunnel: [w137 w151] -> w97
          tunnel: [w136 w151] -> w99
          tunnel: w98 -> [w135 w150]
          tunnel: w96 -> [w134 w149]
          tunnel: w93 -> [w133 _]
          tunnel: [w133 0] -> w92
          frame False {
            n85 = Build Array (concatenate)(w135, w139) -> (w136:T7)
            n86 = Build Array (concatenate)(w134, w138) -> (w137:T7)
          }
          frame True {
            w151 = T7 [] ("Real Matrix")
            n87 = call "MatrixMean.vi"("Real Matrix"=w150) -> ("DevStd Assoluta"=w141:dbl[], "Mean"=w140:dbl[])  [unwired: 8 in, 1 out]
            n88 = call "MatrixMean.vi"("Real Matrix"=w149) -> ("DevStd Assoluta"=w144:dbl[], "Mean"=w145:dbl[])  [unwired: 8 in, 1 out]
            n89 = Build Array (concatenate)(w140, w141) -> (w142:dbl[])
            n90 = Build Array (concatenate)(w145, w144) -> (w143:dbl[])
            n91 = Array To Cluster(array=w142) -> (cluster=→"5 bin mean/std FALL":T1)
            n92 = Array To Cluster(array=w143) -> (cluster=→"5 bin mean/std RISE":T1)
          }
        }
        n93 = feedback-in #1(w99) -> ()
        n94 = feedback-in #2(w97) -> ()
      }
      frame True {
      }
    }
    n95 = local read "stop"() -> (w82:bool)
  }
  n96 = timed-loop {
    tunnel: w36 -> [w295]
    tunnel: w56 -> [w296]
    tunnel: [w298] -> w47
    tunnel: [w299] -> w46
    tunnel: [w284] -> w44
    tunnel: "#Signals" -> [w281]
    timing: w34 -> [_]
    timing-out: [_] -> w33
    shift-right: [w277] -> _
    shift-left: 0 -> [w280]
    tunnel: w14 -> [w276]
    tunnel: w15 -> [w273]
    tunnel: [w271] -> w9
    stop <- "stop" stop-if-true
    n97 = node-c288() -> ()  [unwired: 1 in, 1 out]
    n98 = flat-sequence {
      tunnel: w295 -> [w308]
      tunnel: w296 -> [w309]
      tunnel: "Snapshot" -> [w306]
      tunnel: "Snapshot" -> [w311]
      tunnel: [w310] -> w294
      tunnel: [w311] -> w293
      tunnel: [w306] -> w292
      tunnel: [w310] -> w291
      tunnel: [w307] -> w290
      tunnel: [w307] -> w289
      tunnel: [w305] -> w282
      tunnel: w281 -> [w305]
      tunnel: w280 -> [w304]
      tunnel: [w304] -> w279
      tunnel: w276 -> [w303]
      tunnel: [w303] -> w275
      tunnel: [w302] -> w274
      tunnel: w273 -> [w302]
      tunnel: w294 -> [w332]
      tunnel: w293 -> [w326]
      tunnel: w292 -> [w329]
      tunnel: w291 -> [w328]
      tunnel: w290 -> [w327]
      tunnel: w289 -> [w333]
      tunnel: [w331] -> w288
      tunnel: [w330] -> w287
      tunnel: [w325] -> w286
      tunnel: [w324] -> w283
      tunnel: w282 -> [w323]
      tunnel: w279 -> [w322]
      tunnel: [w322] -> w278
      tunnel: w275 -> [w321]
      tunnel: w274 -> [w320]
      tunnel: [w319] -> w272
      tunnel: [w421] -> w298
      tunnel: [w422] -> w299
      tunnel: w288 -> [w422]
      tunnel: w287 -> [w421]
      tunnel: w286 -> [w419]
      tunnel: [w420] -> w284
      tunnel: w283 -> [w420]
      tunnel: w278 -> [w418]
      tunnel: [w417] -> w277
      tunnel: w272 -> [w416]
      tunnel: [w416] -> w271
      frame #0 {
        n99 = case shown="False" w306 {
          tunnel: [w312 w318] -> w310
          tunnel: w309 -> [w312 w317]
          tunnel: w308 -> [w313 w316]
          tunnel: [w313 w315] -> w307
          frame False {
          }
          frame True {
            n100 = xnode "Read/Write Control"("FPGA VI Reference In"=w316, "error in"=w317, "snapshot"=TRUE) -> ("FPGA VI Reference Out"=w315:refnum<k20>, "error out"=w318:errorcluster)
          }
        }
      }
      frame #1 {
        n101 = flat-sequence {
          tunnel: w333 -> [w342]
          tunnel: w332 -> [w341]
          tunnel: w326 -> [w338]
          tunnel: [w340] -> w336
          tunnel: [w339] -> w335
          tunnel: [w338] -> w334
          tunnel: w323 -> [w337]
          tunnel: [w373] -> w330
          tunnel: w336 -> [w375]
          tunnel: w335 -> [w374]
          tunnel: w334 -> [w372]
          tunnel: [w372] -> w325
          tunnel: [w371] -> w324
          frame #0 {
            n102 = case shown="True" w338 {
              tunnel: w342 -> [w346 w370]
              tunnel: w341 -> [w345 w369]
              tunnel: [w344 w368] -> w339
              tunnel: [w343 w367] -> w340
              tunnel: w337 -> [_ w366]
              frame False {
                n103 = disable-structure shown="Enabled" {
                  disable-tunnel: w346 -> [w353 w356]
                  disable-tunnel: w345 -> [w351 w355]
                  disable-tunnel: [w350 w355] -> w344
                  disable-tunnel: [w347 w356] -> w343
                  frame Disabled {
                    n104 = xnode "Invoke Method"("FPGA VI Reference In"=w353, "error in"=w351, "Number of Elements"=u32 0) -> ("FPGA VI Reference Out"=w349:refnum<k20>, "error out"=w348:errorcluster, "Elements Remaining"=w352:u32)  [unwired: 1 in, 1 out]
                    n105 = xnode "Invoke Method"("FPGA VI Reference In"=w349, "error in"=w348, "Number of Elements"=w352) -> ("FPGA VI Reference Out"=w347:refnum<k20>, "error out"=w350:errorcluster)  [unwired: 1 in, 2 out]
                  }
                  frame Enabled {
                  }
                }
              }
              frame True {
                n106 = Multiply(x=w366, y=u32 1024 ("Number of Elements")) -> (x*y=w360:u32)
                n107 = xnode "Invoke Method"("FPGA VI Reference In"=w370, "error in"=w369, "Number of Elements"=w360, "Timeout (ms)"=-1) -> ("FPGA VI Reference Out"=w363:refnum<k20>, "error out"=w362:errorcluster, "Data"=w365:fxp<+/-,12,12>[])  [unwired: 1 out]
                n108 = To Double Precision Float(number=w365) -> (double precision float=→"N-Signals":dbl[])
                n109 = xnode "Invoke Method"("FPGA VI Reference In"=w363, "error in"=w362, "Number of Elements"=u32 0) -> ("FPGA VI Reference Out"=w367:refnum<k20>, "error out"=w368:errorcluster, "Elements Remaining"=→"Elements Remaining Signal":u32)  [unwired: 1 in, 1 out]
              }
            }
          }
          frame #1 {
            n110 = case shown="False" w372 {
              tunnel: [w377 w380] -> w373
              tunnel: w375 -> [w376 w381]
              tunnel: w374 -> [w377 w379]
              tunnel: [w376 w378] -> w371
              frame False {
              }
              frame True {
                n111 = xnode "Read/Write Control"("FPGA VI Reference In"=w381, "error in"=w379, "snapshot"=FALSE) -> ("FPGA VI Reference Out"=w378:refnum<k20>, "error out"=w380:errorcluster)
              }
            }
          }
        }
        n112 = case shown="True" w329 {
          tunnel: w327 -> [w386 w414]
          tunnel: w328 -> [w385 w415]
          tunnel: [w384 w413] -> w331
          tunnel: w323 -> [_ w401]
          tunnel: w321 -> [w383 w399]
          tunnel: w320 -> [_ w398]
          tunnel: [w383 w396] -> w319
          frame False {
            n113 = disable-structure shown="Enabled" {
              disable-tunnel: w386 -> [w392 _]
              disable-tunnel: w385 -> [w389 w394]
              disable-tunnel: [w388 w394] -> w384
              frame Disabled {
                n114 = xnode "Invoke Method"("FPGA VI Reference In"=w392, "error in"=w389, "Number of Elements"=u32 0) -> ("FPGA VI Reference Out"=w390:refnum<k20>, "error out"=w387:errorcluster, "Elements Remaining"=w391:u32)  [unwired: 1 in, 1 out]
                n115 = xnode "Invoke Method"("FPGA VI Reference In"=w390, "error in"=w387, "Number of Elements"=w391) -> ("error out"=w388:errorcluster)  [unwired: 1 in, 3 out]
              }
              frame Enabled {
              }
            }
          }
          frame True {
            # "256x5"
            # "256x5"
            n116 = Multiply(x=w401, y=u32 1024 ("Number of Elements")) -> (x*y=w405:u32)
            n117 = xnode "Invoke Method"("FPGA VI Reference In"=w414, "error in"=w415, "Number of Elements"=w405, "Timeout (ms)"=-1) -> ("FPGA VI Reference Out"=w409:refnum<k20>, "error out"=w410:errorcluster, "Data"=w412:fxp<+,44,44>[])  [unwired: 1 out]
            n118 = To Double Precision Float(number=w412) -> (double precision float=w411:dbl[])
            n119 = Square Root(x=w411) -> (sqrt(x)=w402:dbl[])
            n120 = xnode "Invoke Method"("FPGA VI Reference In"=w409, "error in"=w410, "Number of Elements"=u32 0) -> ("error out"=w413:errorcluster, "Elements Remaining"=→"Elements Remaining FFT":u32)  [unwired: 1 in, 2 out]
            n121 = call "CleanCompleteFFTArray.vi"("Complete FFT Array"=w402, "FFT Size"=512, "#Signals"=w401) -> ("Second Edge Array"=w400:dbl[], "First Edge Array"=w395:dbl[])  [unwired: 7 in]
            "FALLING First Edge N-FFT" <- w395
            "RISING Second Edge N-FFT" <- w400
            n122 = Build Array (concatenate)(w395, w400) -> (w397:dbl[])
            n123 = RT FIFO Write(0:w399, 1:w397, 3:w398) -> (8:w396:refnum<k33>)  [unwired: 2 in, 3 out]
          }
        }
      }
      frame #2 {
        n124 = case shown="False" w419 {
          tunnel: w418 -> [w423 w427]
          tunnel: [w423 w428] -> w417
          frame False {
          }
          frame True {
            n125 = Decrement(x="tieni premuto per") -> (x-1=w424:i32)
            n126 = Greater Or Equal?(x=w427, y=w424) -> (x >= y?=w426:bool)
            n127 = case shown="True" w426 {
              tunnel: w427 -> [w429 _]
              tunnel: [w430 0] -> w428
              frame False {
                n128 = Increment(x=w429) -> (x+1=w430:i32)
              }
              frame True {
                n129 = local write "Snapshot"(FALSE ("Snapshot")) -> ()
              }
            }
          }
        }
      }
    }
    n130 = node-c288() -> ()  [unwired: 1 in, 1 out]
  }
  n131 = node-c288(w33) -> ()  [unwired: 1 out]
  n132 = Merge Errors(w46, w47) -> (w51:errorcluster)
  n133 = flat-sequence {
    tunnel: w51 -> [w440]
    tunnel: w44 -> [w435]
    tunnel: w9 -> [w433]
    frame #0 {
      n134 = xnode "Invoke Method"("FPGA VI Reference In"=w435, "error in"=w440) -> ("FPGA VI Reference Out"=w437:refnum<k20>, "error out"=w436:errorcluster)
      n135 = RT FIFO Delete(0:w433) -> ()  [unwired: 2 in, 1 out]
      n136 = property on="stop" class="Bool (strict)"("Value"=FALSE ("stop")) -> ()  [unwired: 2 in, 2 out]
      n137 = xnode "Invoke Method"("FPGA VI Reference In"=w437, "error in"=w436) -> ("FPGA VI Reference Out"=w438:refnum<k20>, "error out"=w439:errorcluster)
      n138 = xnode "Close FPGA VI Reference"("FPGA VI Reference In"=w438, "error in"=w439) -> ()  [unwired: 1 out]
    }
  }
